vi "关键参数交互.vi"(9 "量程选择":enum16{"低量程", "高量程", "0-2量程"}(ring), 10 "测量模式(公式)":u16(ring)=1 items=["水样测试"=1, "标样核查"=2, "零点核查"=3, "跨度核查"=4, "空白测试"=5, "平行样"=6, "加标回收"=7], 11 "模型":enum32{"线性", "多项式"}(ring)) -> ()   [LabVIEW 2016, in "斯坦道CODMn.lvlib"]
panel:
  out "x != y?":T1
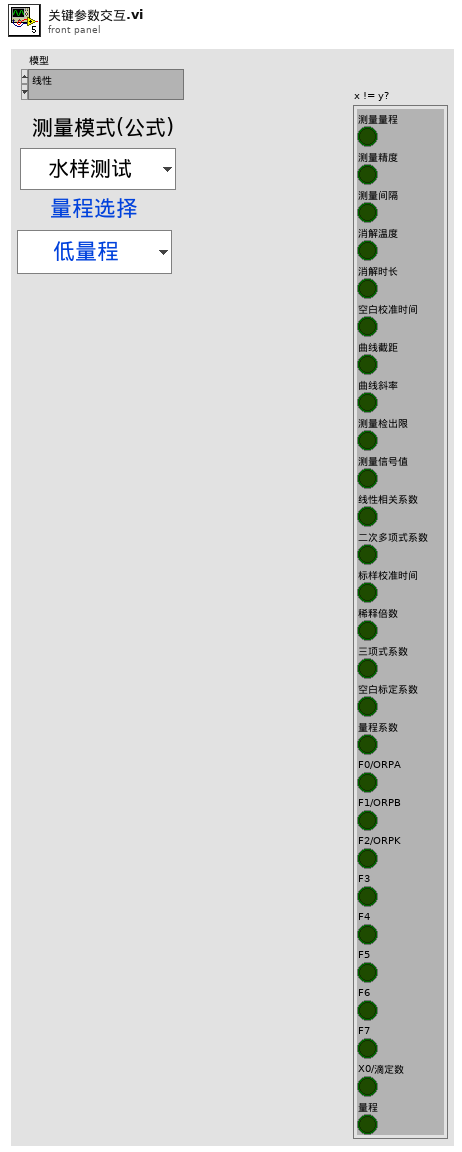
[diagram p1: front panel]
types:
  T1 = cluster{"测量量程":bool, "测量精度":bool, "测量间隔":bool, "消解温度":bool, "消解时长":bool, "空白校准时间":bool, "曲线截距":bool, "曲线斜率":bool, "测量检出限":bool, "测量信号值":bool, "线性相关系数":bool, "二次多项式系数":bool, "标样校准时间":bool, "稀释倍数":bool, "三项式系数":bool, "空白标定系数":bool, "量程系数":bool, "F0/ORPA":bool, "F1/ORPB":bool, "F2/ORPK":bool, "F3":bool, "F4":bool, "F5":bool, "F6":bool, "F7":bool, "X0/滴定数":bool, "量程":bool}
  T2 = cluster{"chose":string, "公式":cluster{"X^2":dbl, "X":dbl, "b":dbl}}
  T3 = cluster{"测量量程":dbl, "测量精度":dbl, "测量间隔":dbl, "消解温度":dbl, "消解时长":dbl, "空白校准时间":timestamp, "曲线截距":dbl, "曲线斜率":dbl, "测量检出限":dbl, "测量信号值":dbl, "线性相关系数":dbl, "二次多项式系数":dbl, "标样校准时间":timestamp, "稀释倍数":dbl, "三项式系数":dbl, "空白标定系数":dbl, "量程系数":dbl, "F0/ORPA":dbl, "F1/ORPB":dbl, "F2/ORPK":dbl, "F3":dbl, "F4":dbl, "F5":dbl, "F6":dbl, "F7":dbl, "X0/滴定数":dbl, "量程":dbl}
  T4 = cluster{"时间标识":timestamp, "设备":string, "日志信息":string, "流程参数":string}
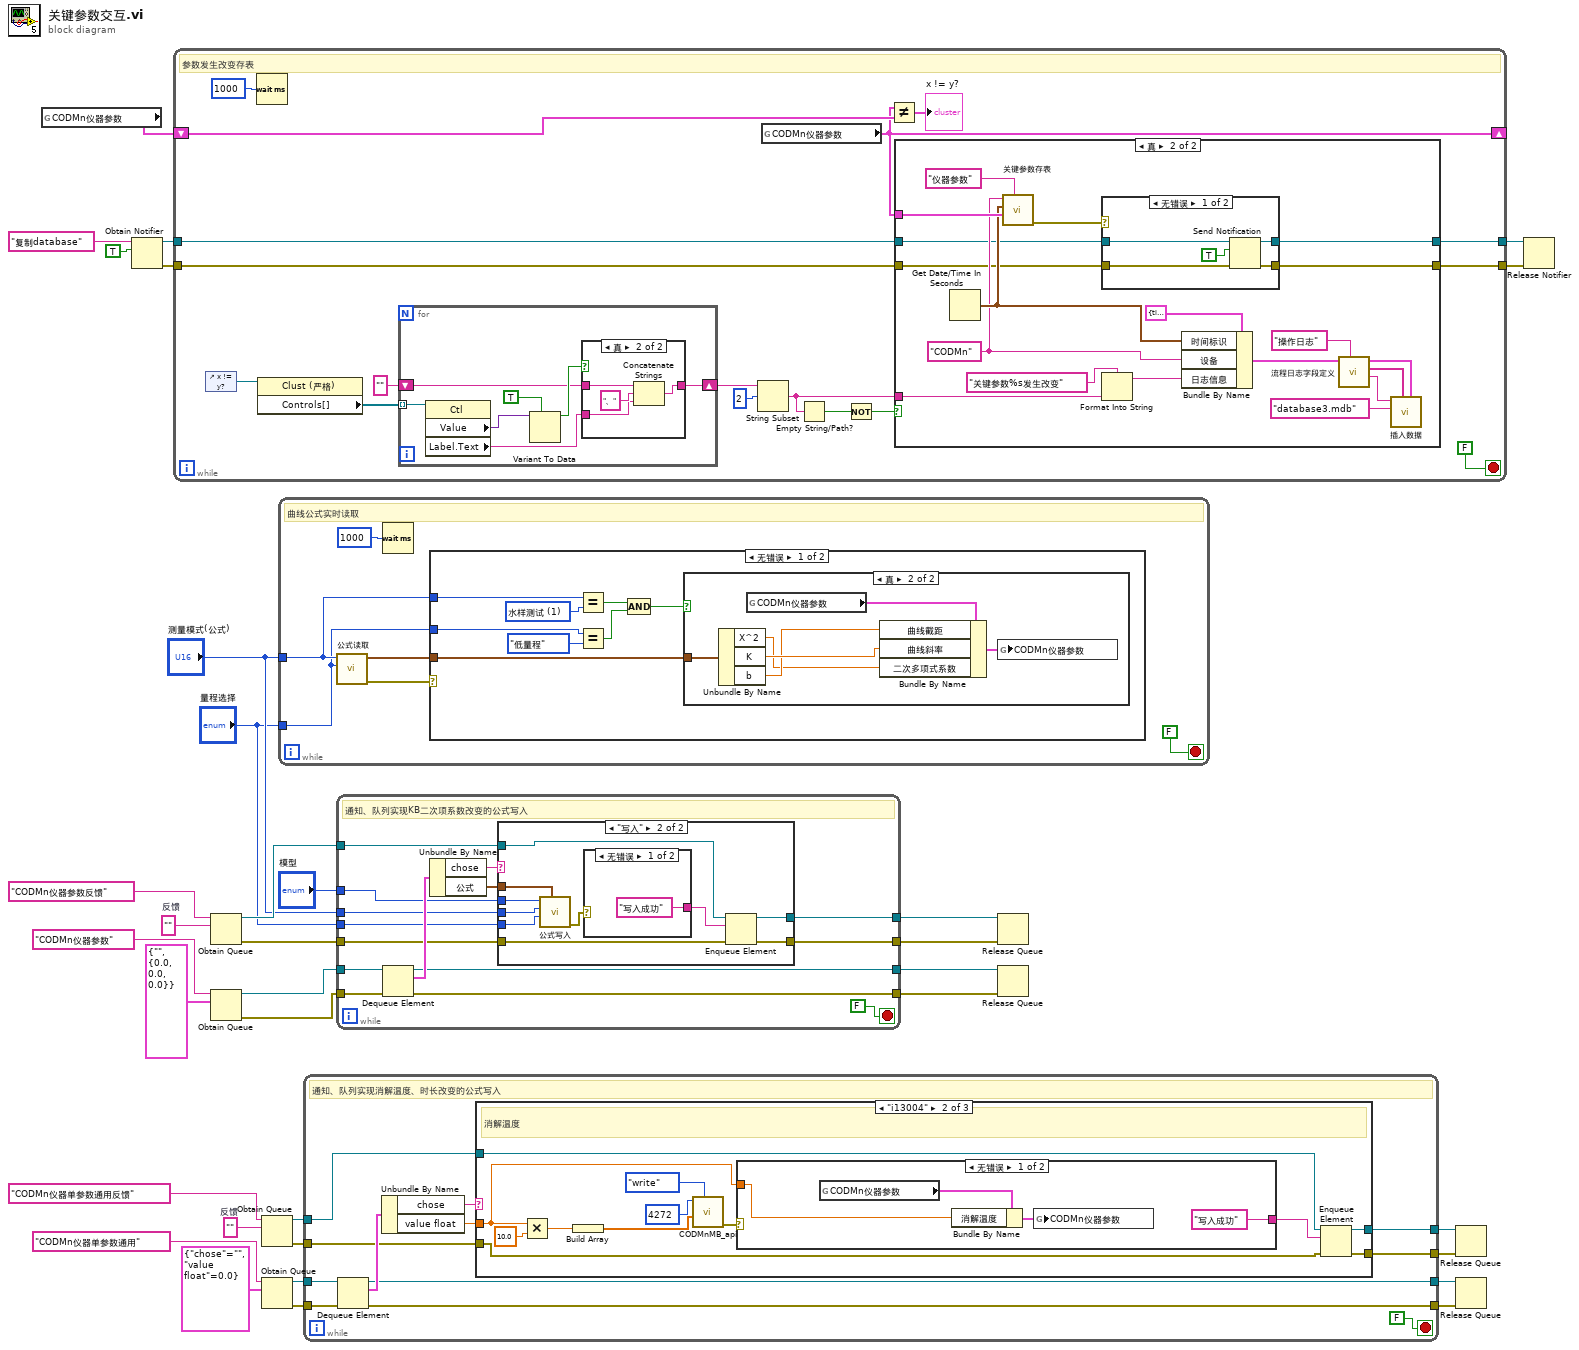
[diagram p0: block diagram]
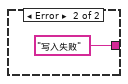
[diagram p3: hidden frame]
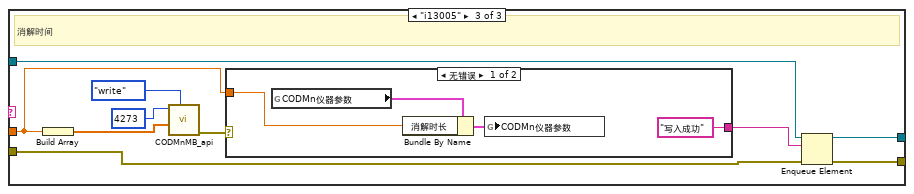
[diagram p4: hidden frame]
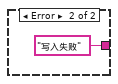
[diagram p5: hidden frame]
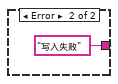
[diagram p9: hidden frame]
diagram:
  w9 = ""  # 反馈
  w25 = ""  # 反馈
  n1 = global read "CODMn断电保存全局变量.vi" "CODMn仪器参数"() -> (w34:T3)
  n2 = Obtain Notifier(name (unnamed)="复制database" ("名称（未命名）"), notification data type=TRUE) -> (notifier out=w19:refnum<notifier>, error out=w18:errorcluster)  [unwired: 2 in, 1 out]
  n3 = while {
    shift-right: [w46] -> _
    shift-left: w34 -> [w49]
    tunnel: w19 -> [w42]
    tunnel: w18 -> [w45]
    tunnel: [w44] -> w17
    tunnel: [w43] -> w16
    stop <- FALSE stop-if-true
    # "参数发生改变存表"
    n4 = control-ref of="x != y?"() -> (w47:refnum<vi>)
    n5 = Wait (ms)(milliseconds to wait=u32 1000 ("等待时间（毫秒）")) -> ()  [unwired: 1 out]
    n6 = property class="Clust (严格)"(reference=w47) -> ("Controls[]"=w37:refnum<vi>[])  [unwired: 1 in, 2 out]
    n7 = for {
      tunnel: w37 -> [w58] mode=indexing
      shift-right: [w52] -> w39
      shift-left: "" -> [w54]
      n8 = property class="Ctl"(reference=w58) -> ("Value"=w56:variant, "Label.Text"=w53:string)  [unwired: 1 in, 2 out]
      n9 = Variant To Data(type=TRUE, Variant=w56) -> (data=w55:bool)  [unwired: 1 in, 1 out]
      n10 = case shown="真" w55 {
        tunnel: w54 -> [w59 w63]
        tunnel: w53 -> [_ w60]
        tunnel: [w59 w62] -> w52
        frame False {
        }
        frame True {
          n11 = Concatenate Strings(w63, "、", w60) -> (w62:string)
        }
      }
    }
    n12 = String Subset(string=w39, offset (0)=2 ("偏移量(0)")) -> (substring=w35:string)  [unwired: 1 in]
    n13 = global read "CODMn断电保存全局变量.vi" "CODMn仪器参数"() -> (w46:T3)
    n14 = Empty String/Path?(string/path=w35) -> (empty?=w41:bool)
    n15 = Not(x=w41) -> (.not. x?=w36:bool)
    n16 = Not Equal?(x=w46, y=w49) -> (x != y?=→"x != y?":T1)
    n17 = case shown="真" w36 {
      tunnel: w46 -> [_ w83]
      tunnel: w35 -> [_ w78]
      tunnel: w45 -> [w65 w69]
      tunnel: [w64 w68] -> w44
      tunnel: [w65 w67] -> w43
      tunnel: w42 -> [w64 w66]
      frame False {
      }
      frame True {
        w80 = "CODMn" ("仪器名称")
        n18 = Get Date/Time In Seconds() -> (seconds since 1Jan1904=w81:timestamp)
        n19 = call "关键参数存表.vi"("table"="仪器参数", "仪器参数"=w83, "datatime"=w81, "仪器名称"=w80) -> ("error out"=w70:errorcluster)  [unwired: 7 in]
        n20 = case shown="无错误" w70 {
          tunnel: w66 -> [w89 w91]
          tunnel: w69 -> [w88 w90]
          tunnel: [w86 w91] -> w68
          tunnel: [w85 w90] -> w67
          frame No Error {
            n21 = Send Notification(notification=TRUE ("通知"), notifier=w89, error in (no error)=w88) -> (notifier out=w86:refnum<notifier>, error out=w85:errorcluster)
          }
          frame Error {
          }
        }
        n22 = Format Into String(format string="关键参数%s发生改变" ("格式字符串"), w78) -> (resulting string=w77:string)  [unwired: 2 in, 1 out]
        n23 = Bundle By Name(cluster=T4 {"时间标识"=timestamp(0 s since 1904-01-01), "设备"="", "日志信息"="", "流程参数"=""} ("data in"), "时间标识"=w81, "设备"=w80, "日志信息"=w77) -> (w71:T4)
        n24 = call "流程日志字段定义.vi"("table输入"="操作日志", "data in"=w71) -> ("table输出"=w74:string, "columns"=w75:string[], "data out"=w76:T4)  [unwired: 7 in]
        n25 = call "插入数据.vi"("data"=w76, "columns"=w75, "database"="database3.mdb", "table"=w74) -> ()  [unwired: 7 in, 1 out]
      }
    }
  }
  n26 = Obtain Queue(name (unnamed)="CODMn仪器参数反馈" ("名称（未命名）"), element data type=w25) -> (queue out=w26:refnum<queue>, error out=w24:errorcluster)  [unwired: 3 in, 1 out]
  n27 = Obtain Queue(name (unnamed)="CODMn仪器参数" ("名称（未命名）"), element data type=T2 {"chose"="", "公式"={"X^2"=0.0, "X"=0.0, "b"=0.0}}) -> (queue out=w33:refnum<queue>, error out=w32:errorcluster)  [unwired: 3 in, 1 out]
  n28 = Obtain Queue(name (unnamed)="CODMn仪器单参数通用反馈" ("名称（未命名）"), element data type=w9) -> (queue out=w8:refnum<queue>, error out=w10:errorcluster)  [unwired: 3 in, 1 out]
  n29 = Obtain Queue(name (unnamed)="CODMn仪器单参数通用" ("名称（未命名）"), element data type=cluster{"chose":string, "value float":dbl} {"chose"="", "value float"=0.0}) -> (queue out=w1:refnum<queue>, error out=w2:errorcluster)  [unwired: 3 in, 1 out]
  n30 = while {
    tunnel: "测量模式(公式)" -> [w94]
    tunnel: "量程选择" -> [w93]
    stop <- FALSE stop-if-true
    # "曲线公式实时读取"
    n31 = call "公式读取.vi"("量程选择"=w93, "测量模式(公式)"=w94) -> ("error out"=w92:errorcluster, "方程系数"=w95:cluster{"K":dbl, "b":dbl, "X^2":dbl})  [unwired: 8 in]
    n32 = Wait (ms)(milliseconds to wait=u32 1000 ("等待时间（毫秒）")) -> ()  [unwired: 1 out]
    n33 = case shown="无错误" w92 {
      tunnel: w94 -> [w105 _]
      tunnel: w95 -> [w101 _]
      tunnel: w93 -> [w100 _]
      frame No Error {
        w99 = u16 1 items=["水样测试"=1, "标样核查"=2, "零点核查"=3, "跨度核查"=4, "空白测试"=5, "平行样"=6, "加标回收"=7] ("测量模式(公式)")
        n34 = Equal?(x=w105, y=w99) -> (x = y?=w104:bool)
        n35 = Equal?(x=w100, y=enum16{"低量程", "高量程", "0-2量程"}."低量程" ("量程选择")) -> (x = y?=w103:bool)
        n36 = Compound Arithmetic op=AND ("复合运算")(w104, w103) -> (w102:bool)
        n37 = case shown="真" w102 {
          tunnel: w101 -> [_ w111]
          frame False {
          }
          frame True {
            n38 = Unbundle By Name(w111) -> ("X^2"=w108:dbl, "K"=w110:dbl, "b"=w109:dbl)
            n39 = global read "CODMn断电保存全局变量.vi" "CODMn仪器参数"() -> (w107:T3)
            n40 = Bundle By Name(cluster=w107, "曲线截距"=w109, "曲线斜率"=w110, "二次多项式系数"=w108) -> (w106:T3)
            n41 = global write "CODMn断电保存全局变量.vi" "CODMn仪器参数"(w106) -> ()
          }
        }
      }
      frame Error {
      }
    }
  }
  n42 = while {
    tunnel: w1 -> [w122]
    tunnel: w2 -> [w121]
    tunnel: [w117] -> w5
    tunnel: [w116] -> w6
    tunnel: w8 -> [w115]
    tunnel: w10 -> [w114]
    tunnel: [w113] -> w11
    tunnel: [w112] -> w12
    stop <- FALSE stop-if-true
    # "通知、队列实现消解温度、时长改变的公式写入"
    n43 = Dequeue Element(queue=w122, error in (no error)=w121) -> (queue out=w117:refnum<queue>, element=w120:cluster{"chose":string, "value float":dbl}, error out=w116:errorcluster)  [unwired: 1 in, 1 out]
    n44 = Unbundle By Name(w120) -> ("chose"=w119:string, "value float"=w118:dbl)
    n45 = case shown="\"i13004\"" w119 {
      tunnel: w118 -> [_ w126 w143]
      tunnel: w115 -> [w125 w137 w152]
      tunnel: w114 -> [w124 w135 w148]
      tunnel: [w125 w134 w150] -> w113
      tunnel: [w124 w133 w149] -> w112
      frame "假", Default {
      }
      frame "i13004" {
        # "消解温度"
        n46 = Multiply(x=w126, y=10.0) -> (x*y=w129:dbl)
        n47 = Build Array(w129) -> (w128:dbl[])
        n48 = call "CODMnMB_api.vi"("STEP"=enum16{"open", "read", "write", "close"}."write", "values"=w128, "starting address"=u16 4272) -> ("error out"=w127:errorcluster)  [unwired: 6 in, 2 out]
        n49 = case shown="无错误" w127 {
          tunnel: ["写入成功" ("消息") "写入失败" ("消息")] -> w136
          tunnel: w126 -> [w138 _]
          frame No Error {
            n50 = global read "CODMn断电保存全局变量.vi" "CODMn仪器参数"() -> (w140:T3)
            n51 = Bundle By Name(cluster=w140, "消解温度"=w138) -> (w139:T3)
            n52 = global write "CODMn断电保存全局变量.vi" "CODMn仪器参数"(w139) -> ()
          }
          frame Error {
          }
        }
        n53 = Enqueue Element(queue=w137, element=w136, error in (no error)=w135) -> (queue out=w134:refnum<queue>, error out=w133:errorcluster)  [unwired: 1 in, 1 out]
      }
      frame "i13005" {
        # "消解时间"
        n54 = Build Array(w143) -> (w145:dbl[])
        n55 = call "CODMnMB_api.vi"("STEP"=enum16{"open", "read", "write", "close"}."write", "values"=w145, "starting address"=u16 4273) -> ("error out"=w144:errorcluster)  [unwired: 6 in, 2 out]
        n56 = case shown="无错误" w144 {
          tunnel: ["写入成功" ("消息") "写入失败" ("消息")] -> w151
          tunnel: w143 -> [w154 _]
          frame No Error {
            n57 = global read "CODMn断电保存全局变量.vi" "CODMn仪器参数"() -> (w155:T3)
            n58 = Bundle By Name(cluster=w155, "消解时长"=w154) -> (w153:T3)
            n59 = global write "CODMn断电保存全局变量.vi" "CODMn仪器参数"(w153) -> ()
          }
          frame Error {
          }
        }
        n60 = Enqueue Element(queue=w152, element=w151, error in (no error)=w148) -> (queue out=w150:refnum<queue>, error out=w149:errorcluster)  [unwired: 1 in, 1 out]
      }
    }
  }
  n61 = while {
    tunnel: w33 -> [w171]
    tunnel: w32 -> [w170]
    tunnel: [w166] -> w29
    tunnel: [w165] -> w28
    tunnel: w26 -> [w164]
    tunnel: w24 -> [w163]
    tunnel: [w162] -> w23
    tunnel: [w161] -> w22
    tunnel: "模型" -> [w160]
    tunnel: "测量模式(公式)" -> [w159]
    tunnel: "量程选择" -> [w158]
    stop <- FALSE stop-if-true
    # "通知、队列实现KB二次项系数改变的公式写入"
    n62 = Dequeue Element(queue=w171, error in (no error)=w170) -> (queue out=w166:refnum<queue>, element=w169:T2, error out=w165:errorcluster)  [unwired: 1 in, 1 out]
    n63 = Unbundle By Name(w169) -> ("chose"=w168:string, "公式"=w167:cluster{"X^2":dbl, "X":dbl, "b":dbl})
    n64 = case shown="\"写入\"" w168 {
      tunnel: w167 -> [_ w179]
      tunnel: w164 -> [w174 w184]
      tunnel: w163 -> [w173 w182]
      tunnel: [w174 w181] -> w162
      tunnel: [w173 w180] -> w161
      tunnel: w160 -> [_ w177]
      tunnel: w159 -> [_ w176]
      tunnel: w158 -> [_ w175]
      frame "假", Default {
      }
      frame "写入" {
        n65 = call "公式写入.vi"("公式"=w179, "量程选择"=w175, "测量模式(公式)"=w176, "模型"=w177) -> ("error out"=w178:errorcluster)  [unwired: 7 in]
        n66 = case shown="无错误" w178 {
          tunnel: ["写入成功" ("消息") "写入失败" ("消息")] -> w183
          frame No Error {
          }
          frame Error {
          }
        }
        n67 = Enqueue Element(queue=w184, element=w183, error in (no error)=w182) -> (queue out=w181:refnum<queue>, error out=w180:errorcluster)  [unwired: 1 in, 1 out]
      }
    }
  }
  n68 = Release Queue(queue=w23, error in (no error)=w22) -> ()  [unwired: 1 in, 3 out]
  n69 = Release Queue(queue=w29, error in (no error)=w28) -> ()  [unwired: 1 in, 3 out]
  n70 = Release Queue(queue=w11, error in (no error)=w12) -> ()  [unwired: 1 in, 3 out]
  n71 = Release Queue(queue=w5, error in (no error)=w6) -> ()  [unwired: 1 in, 3 out]
  n72 = Release Notifier(notifier=w17, error in (no error)=w16) -> ()  [unwired: 1 in, 3 out]
